vi "Tx Core.vi"(0 "duc parameters":T1[](array[typedef]) {"frequency shift" format="%#.48g"}, 1 "tx.reset":bool=TRUE, 5 "tx.samples to generate":u32, 7 "tx.abort":bool, 9 "tx.stream enable":bool[](array[boolean])=[FALSE, FALSE], 11 "tx.start trigger":bool) -> (4 "tx.state":T4, 6 "tx.samples processed":u32, 8 "tx.number of fifo underflows":u32, 10 "tx 0.number of IQ data overflows":u64, 14 "tx.dsp reset done":bool, 15 "tx 1.number of IQ data overflows":u64)   [LabVIEW 2023]
uses:
  <vilib>/eio/EIONode/EIONode.xnode
  <vilib>/rvi/eio/common/nirviEmuTemplateMethod_errors.vi
  <instrlib>/niUSRP/Reference FPGA/USRPRIO Sample VIs/FPGA/SubVIs/Stream Control State.ctl
  <instrlib>/_niInstr/DSP/v1/Shared/Public/IQ Impairments.ctl
  <instrlib>/_niInstr/DSP/v1/Shared/Public/IQ Gain.ctl
  <instrlib>/niUSRP/Reference FPGA/USRPRIO Sample VIs/FPGA/SubVIs/DUC Parameters.ctl
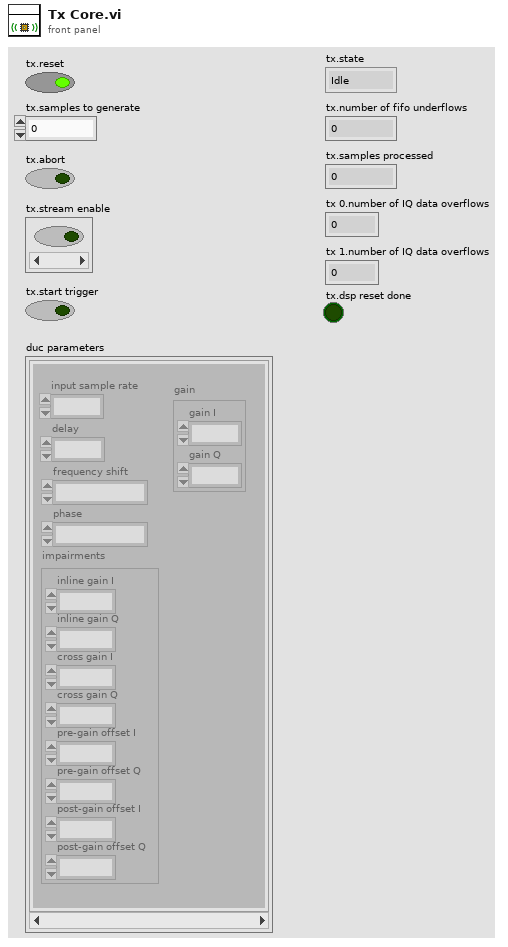
[diagram p1: front panel]
types:
  T1 = typedef "DUC Parameters.ctl" = cluster{"frequency shift":fxp<+/-,48,0>, "impairments":T2, "phase":fxp<+/-,21,0>, "input sample rate":fxp<+,48,1>, "gain":T3, "delay":fxp<+/-,18,0>}
  T2 = typedef "niInstr DSP v1 Shared.lvlib/IQ Impairments.ctl" = cluster{"inline gain I":fxp<+/-,18,1>, "inline gain Q":fxp<+/-,18,1>, "cross gain I":fxp<+/-,18,1>, "cross gain Q":fxp<+/-,18,1>, "pre-gain offset I":fxp<+/-,18,1>, "pre-gain offset Q":fxp<+/-,18,1>, "post-gain offset I":fxp<+/-,18,1>, "post-gain offset Q":fxp<+/-,18,1>}
  T3 = typedef "niInstr DSP v1 Shared.lvlib/IQ Gain.ctl" = cluster{"gain I":fxp<+/-,24,3>, "gain Q":fxp<+/-,24,3>}
  T4 = typedef "Stream Control State.ctl" = enum16{"Idle", "Active"}
  T5 = typedef "niInstr DSP v1 Shared.lvlib/IQ Data.ctl" = cluster{"I":fxp<+/-,18,1>, "Q":fxp<+/-,18,1>, "overflow":bool}
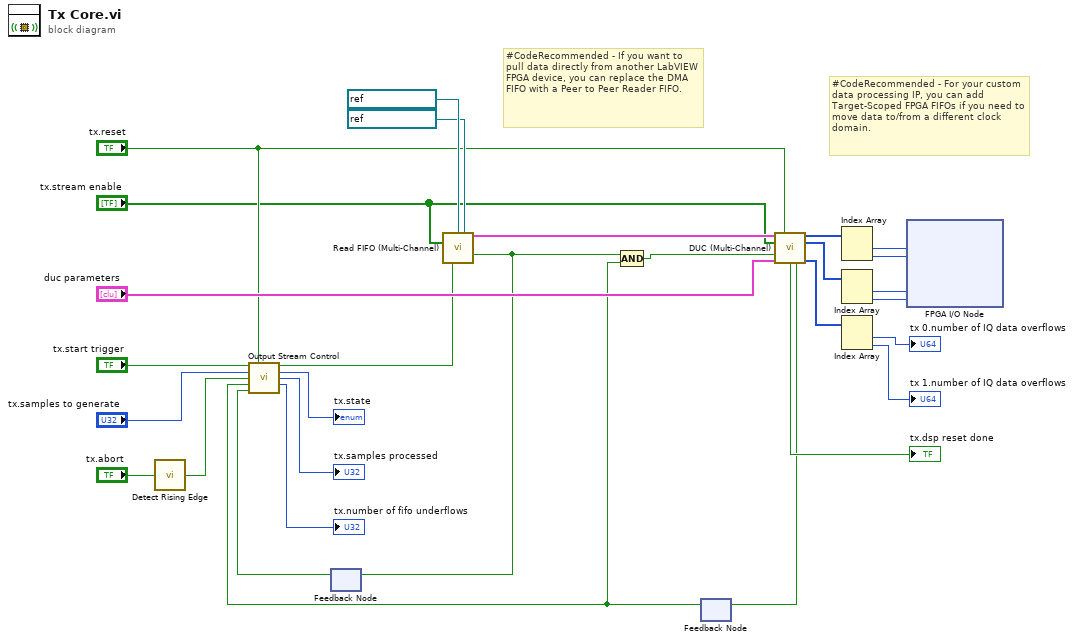
[diagram p0: block diagram]
diagram:
  # "#CodeRecommended - For your custom data processing IP, you can add Target-Scoped FPGA FIFOs if you need to move data to/from a different clock domain."
  # "#CodeRecommended - If you want to pull data directly from another LabVIEW FPGA device, you can replace the DMA FIFO with a Peer to Peer Reader FIFO."
  n1 = call <instrlib>:"Detect Rising Edge.vi"("signal"="tx.abort") -> ("edge detected"=w10:bool)  [unwired: 14 in]
  n2 = feedback #1() -> (w6:bool)  [unwired: 1 in]
  n3 = feedback #2() -> (w8:bool)  [unwired: 1 in]
  n4 = call <instrlib>:"Output Stream Control.vi"("start trigger"="tx.start trigger", "reset"="tx.reset", "burst size"="tx.samples to generate", "abort"=w10, "ready to read stream (T)"=w8, "fifo output valid"=w6) -> ("read stream"=w11:bool, "state"=→"tx.state":T4, "samples processed"=→"tx.samples processed":u32, "number of underflows"=→"tx.number of fifo underflows":u32)  [unwired: 5 in, 1 out]
  n5 = call <instrlib>:"Read FIFO (Multi-Channel).vi"("FIFO 0"=refnum<k21> "Tx Stream 0" ("fifo"), "FIFO 1"=refnum<k21> "Tx Stream 1" ("fifo"), "enabled"="tx.stream enable", "ready for output"=w11) -> ("data out"=w12:T5[], "output valid"=w1:bool)  [unwired: 10 in]
  n6 = feedback-in #1(w1) -> ()
  n7 = Compound Arithmetic op=AND(w1, w8) -> (w26:bool)
  n8 = call <instrlib>:"DUC (Multi-Channel).vi"("data in"=w12, "reset"="tx.reset", "enabled"="tx.stream enable", "input valid"=w26, "DUC Parameters"="duc parameters") -> ("I data out"=w17:i16[], "Q data out"=w19:i16[], "dsp reset done"=→"tx.dsp reset done":bool, "ready for input"=w13:bool, "number of overflows"=w16:u64[])  [unwired: 5 in, 1 out]
  n9 = feedback-in #2(w13) -> ()
  n10 = Index Array(array=w17) -> (element #1=w18:i16, element #2=w21:i16)  [unwired: 2 in]
  n11 = Index Array(array=w19) -> (element #1=w22:i16, element #2=w23:i16)  [unwired: 2 in]
  n12 = Index Array(array=w16) -> (element #1=→"tx 0.number of IQ data overflows":u64, element #2=→"tx 1.number of IQ data overflows":u64)  [unwired: 2 in]
  n13 = xnode "FPGA I/O Node"("RF 0/Tx/I"=w18, "RF 1/Tx/I"=w21, "RF 0/Tx/Q"=w22, "RF 1/Tx/Q"=w23) -> ()  [unwired: 4 in, 4 out]
